vi "SyringePumpMain.vi"() -> ()   [LabVIEW 2016]
uses:
  <extravilib>/ChannelInstances/Tag-bool/Read With Abort.vi
  <extravilib>/ChannelInstances/Tag-bool/Write.vi
  <extravilib>/ChannelInstances/Tag-bool/Write With Abort.vi
  <extravilib>/ChannelInstances/Tag-bool/Instantiate.vi
  <extravilib>/ChannelInstances/Tag-bool/EndpointRead.vi
  <extravilib>/ChannelInstances/Tag-bool/Endpoint.vi
  <instrlib>/KD Scientific Legato 2XX Series/KD Scientific Legato 2XX Series.lvlib
  <extravilib>/ChannelInstances/Tag-bool.lvlib
panel:
  in  "Pause loop":bool
  in  "Infusion Rate \nUnits":u32(ring)=3 items=["ml/hr", "ml/min", "ul/hr", "ul/min", "ul/sec", "nl/sec"]
  out "Output infusion rate":string
  in  "Set infusion rate":bool
  in  "Infusion rate":dbl=2.0
  out "Output infusion volume":string
  in  "Set infusion volume":bool
  in  "Infusion \nVolume":i32=100
  in  "Infusion \nVolume unit":u16(ring) items=["µL", "nL", "mL"]
  out "Time remaining":dbl format="%<%H:%M:%S>t"
  out "Target reached?":bool
  out "Infusing?":bool
  out "Del. volume":string="0 nl"
  out "Path":path
  in  "Withdraw Rate \nUnits":u32(ring)=3 items=["ml/hr", "ml/min", "ul/hr", "ul/min", "ul/sec", "nl/sec"]
  out "Output withdraw rate":string
  in  "Set withdraw rate":bool
  in  "Withdraw rate":dbl=2.0
  out "Output withdraw volume":string
  in  "Set withdraw volume":bool
  in  "Withdraw \nVolume":i32=100
  in  "Withdraw \nVolume unit":u16(ring) items=["µL", "nL", "mL"]
  in  "Infuse":bool=TRUE
  in  "Withdraw":bool
  in  "Save Configuration":bool
  in  "Reset":bool
  in  "Start/Stop":bool
  in  "stop":bool
  in  "Syringe Volume Unit":u16(ring) items=["µL", "nL", "mL"]
  out "Output syringe volume":string
  in  "Set syringe volume":bool
  in  "Syringe Volume":i32=30 min=0 max=100 step=1
  out "Output force":string
  in  "Set force":bool
  in  "Current Force":i32=30 min=0 max=100 step=1
  out "Output syringe diameter":string
  in  "Set syringe diameter":bool
  in  "Syringe Diameter (mm)":dbl=4.86 min=0.01 max=49.99 step=0.01 format="%.2g"
  out "VISA resource":refnum<visa-resource-name>
  # "Syringe Volume"
  # "Force"
  # "Infusion rate"
  # "Infusion volume"
  # "Infusing:"
  # "Time remaining:"
  # "Volume delivered:"
  # "Target reached:"
  # "Withdraw rate"
  # "Withdraw volume"
  # "Syringe Diameter"
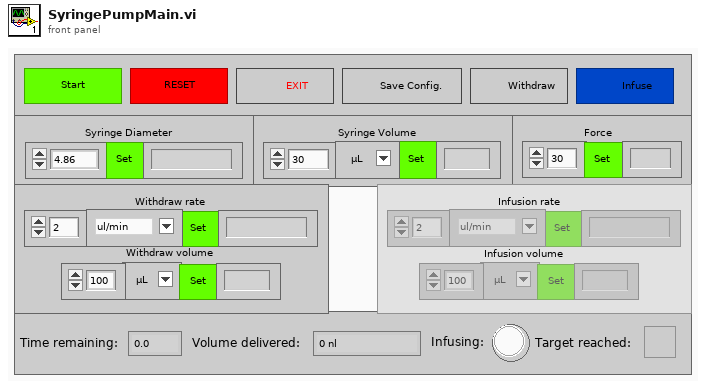
[diagram p1: front panel]
types:
  T1 = enum8{"Enabled", "Disabled", "Disabled and Grayed Out"}
  T2 = enum32{"invalid app kind", "Development System", "Run Time System", "Student Edition", "Embedded LabVIEW", "Evaluation", "Custom"}
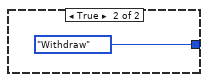
[diagram p4: hidden frame]
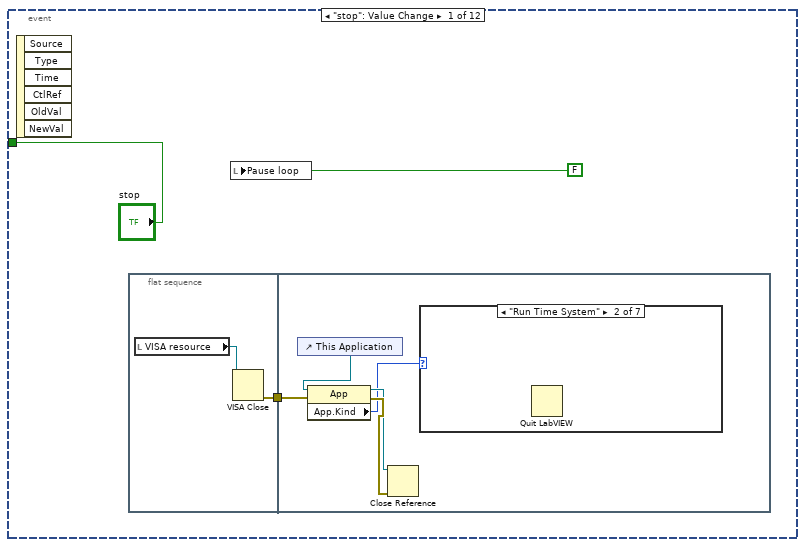
[diagram p6: hidden frame]
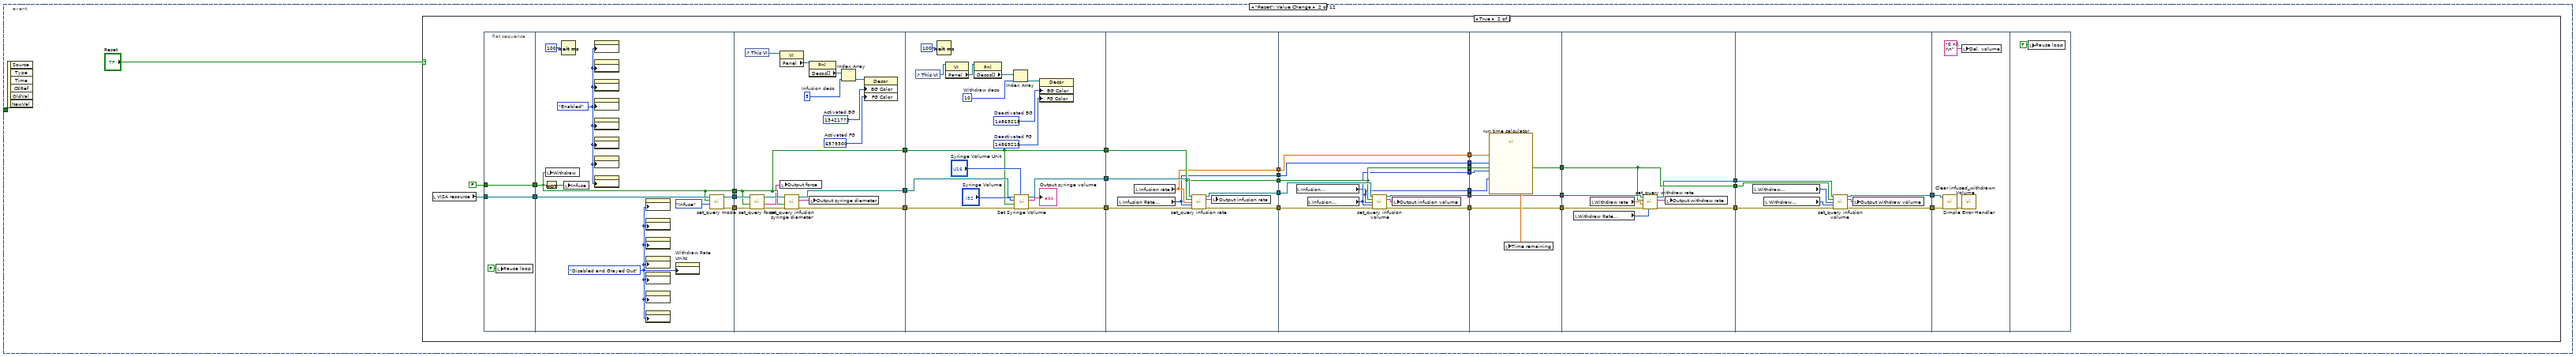
[diagram p13: hidden frame]
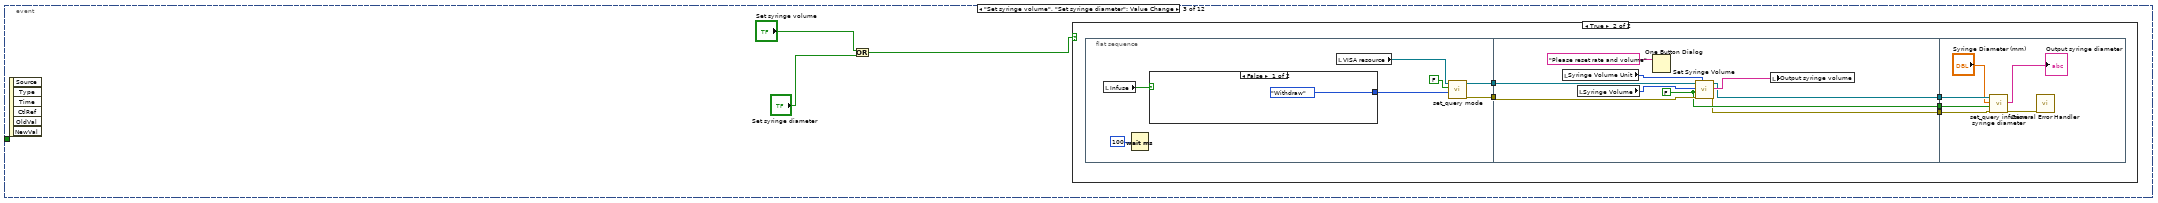
[diagram p15: hidden frame]
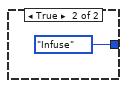
[diagram p17: hidden frame]
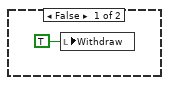
[diagram p18: hidden frame]
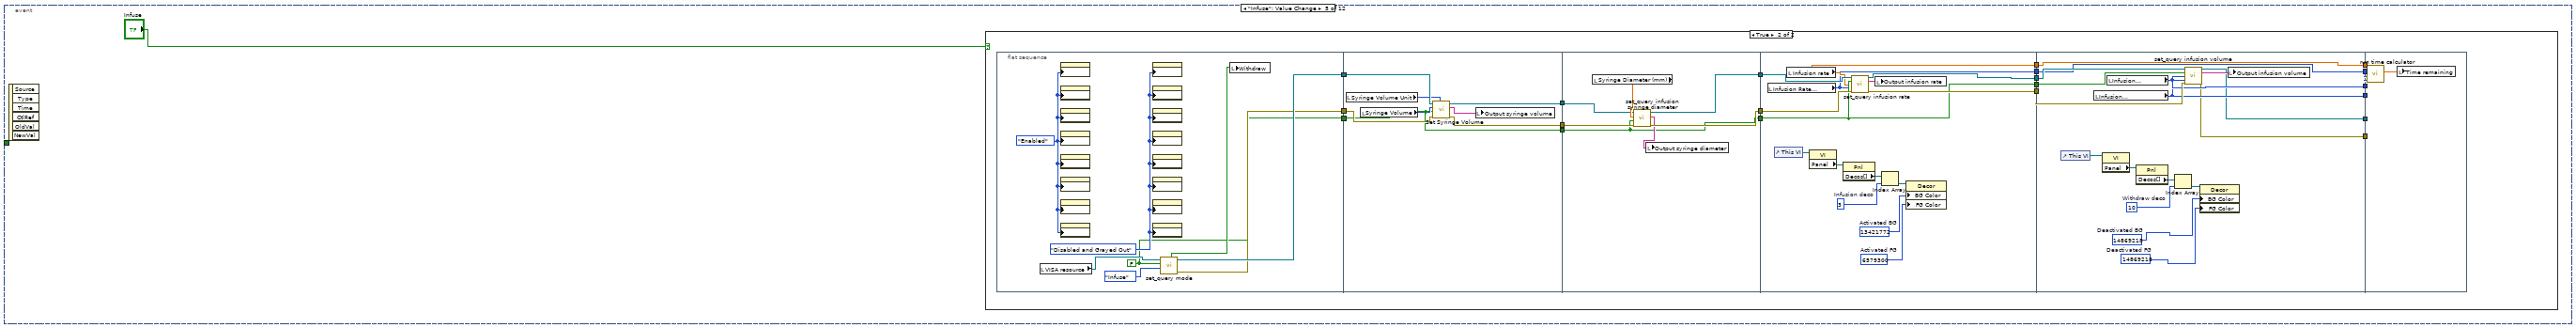
[diagram p19: hidden frame]
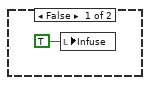
[diagram p20: hidden frame]
diagram:
  n1 = flat-sequence "Initialization sequence" {
    tunnel: [w39] -> w11
    tunnel: [w50] -> w32
    tunnel: [w73] -> w31
    tunnel: [w60] -> w30
    tunnel: [w72] -> w28
    tunnel: [w63] -> w26
    tunnel: [w55] -> w22
    tunnel: [w54] -> w14
    tunnel: [w53] -> w12
    tunnel: w11 -> [w51]
    tunnel: w32 -> [w99]
    tunnel: w31 -> [w96]
    tunnel: w30 -> [w103]
    tunnel: [w103] -> w29
    tunnel: w28 -> [w102]
    tunnel: [w102] -> w27
    tunnel: w26 -> [w101]
    tunnel: [w98] -> w25
    tunnel: [w97] -> w24
    tunnel: [w92] -> w23
    tunnel: w22 -> [w92]
    tunnel: w14 -> [w85]
    tunnel: [w84] -> w13
    tunnel: w12 -> [w84]
    tunnel: w29 -> [w118]
    tunnel: [w120] -> w38
    tunnel: w27 -> [w117]
    tunnel: [w116] -> w36
    tunnel: [w113] -> w35
    tunnel: w25 -> [w112]
    tunnel: w24 -> [w111]
    tunnel: w23 -> [w110]
    tunnel: [w110] -> w21
    tunnel: w13 -> [w104]
    tunnel: w38 -> [w129]
    tunnel: [w126] -> w37
    tunnel: w36 -> [w128]
    tunnel: w35 -> [w127]
    tunnel: [w127] -> w34
    tunnel: [w125] -> w33
    tunnel: w21 -> [w122]
    tunnel: [w122] -> w20
    tunnel: w37 -> [w138]
    tunnel: w34 -> [w135]
    tunnel: w33 -> [w139]
    tunnel: w20 -> [w141]
    tunnel: [w137] -> w19
    tunnel: [w140] -> w18
    tunnel: [w135] -> w17
    tunnel: [w141] -> w16
    tunnel: w19 -> [w146]
    tunnel: w18 -> [w147]
    tunnel: [w150] -> w10
    tunnel: w17 -> [w145]
    tunnel: w16 -> [w151]
    tunnel: [w145] -> w7
    tunnel: [w148] -> w4
    tunnel: [w151] -> w2
    tunnel: w10 -> [w158]
    tunnel: [w157] -> w8
    tunnel: w7 -> [w156]
    tunnel: [w156] -> w6
    tunnel: [w155] -> w5
    tunnel: w4 -> [w154]
    tunnel: [w153] -> w3
    tunnel: w2 -> [w153]
    tunnel: [w167] -> w9
    tunnel: w8 -> [w168]
    tunnel: w6 -> [w166]
    tunnel: w5 -> [w165]
    tunnel: w3 -> [w163]
    tunnel: [w163] -> w1
    tunnel: w9 -> [w177]
    tunnel: w1 -> [w176]
    frame #0 {
      n2 = control-ref of="This Application"() -> (w44:refnum<vi>)
      n3 = property class="App"(reference=w44) -> (reference out=w42:refnum<vi>, error out=w41:errorcluster, "App.Kind"=w43:T2)  [unwired: 1 in]
      n4 = control-ref of="This VI"() -> (w40:refnum<vi>)
      n5 = Close Reference(reference=w42, error in (no error)=w41) -> ()  [unwired: 1 out]
      n6 = invoke class="VI" method="Default Vals.Reinit All"(reference=w40) -> ()  [unwired: 2 in, 3 out]
      n7 = case shown="\"Run Time System\"" w43 {
        tunnel: [w45 w47 _ _ _ _ _] -> w39
        tunnel: w40 -> [w46 _ _ _ _ _ _]
        frame "Development System" {
          n8 = property class="VI"(reference=w46) -> ("Path"=w45:path)  [unwired: 1 in, 2 out]
        }
        frame "Run Time System" {
          n9 = call <userlib>:"Application Directory__ogtk.vi"() -> ("Application Directory (+ Relative)"=w49:path)  [unwired: 1 in]
          n10 = Build Path(base path=w49, name or relative path="Syringe Pump Controller\\") -> (appended path=w47:path)
        }
        frame "Student Edition" {
        }
        frame "Embedded LabVIEW" {
        }
        frame "Evaluation" {
        }
        frame "Custom" {
        }
        frame "invalid app kind" {
        }
      }
    }
    frame #1 {
      n11 = call "Config Reader.vi"("Path"=w51) -> ("Withdraw rate"=w56:dbl, "Withdraw \nVolume unit"=w58:u16, "Withdraw \nVolume"=w59:i32, "Default Current Force"=w72:i32, "Default Volume unit"=w69:u16, "Mode"=w65:string, "Withdraw Rate \nUnits"=w57:u32, "Default Syringe Volume Unit"=w66:u16, "Default Flow Rate Units (1:ml/min)"=w70:u32, "Default Volume"=w68:i32, "VISA Refnum out"=w50:refnum<visa-resource-name>, "Default Infusion rate"=w71:dbl, "Default Syringe Volume"=w67:i32, "Default Syringe Diameter (mm)"=w60:dbl, "error out"=w73:errorcluster)  [unwired: 4 in]
      n12 = local write "Current Force"(w72) -> ()
      n13 = local write "Infusion Rate \nUnits"(w70) -> ()
      n14 = local write "Infusion rate"(w71) -> ()
      n15 = local write "Syringe Diameter (mm)"(w60) -> ()
      n16 = local write "Syringe Volume"(w67) -> ()
      n17 = local write "Syringe Volume Unit"(w66) -> ()
      n18 = local write "Infusion \nVolume"(w68) -> ()
      n19 = local write "Infusion \nVolume unit"(w69) -> ()
      n20 = local write "Withdraw \nVolume"(w59) -> ()
      n21 = local write "Withdraw \nVolume unit"(w58) -> ()
      n22 = local write "Withdraw rate"(w56) -> ()
      n23 = local write "Withdraw Rate \nUnits"(w57) -> ()
      n24 = property class="Instr"(reference=w50, "General Settings:Timeout Value"=u32 10000) -> ()  [unwired: 1 in, 2 out]
      n25 = Equal?(x=w65, y="Infuse") -> (x = y?=w55:bool)
      n26 = case shown="True" w55 {
        tunnel: [enum16{"Withdraw", "Infuse"}."Withdraw" ("Mode Selector") enum16{"Withdraw", "Infuse"}."Infuse" ("Mode Selector")] -> w63
        tunnel: [T1."Disabled and Grayed Out" ("Disabled") T1."Enabled" ("Disabled")] -> w62
        tunnel: [T1."Enabled" ("Disabled") T1."Disabled and Grayed Out" ("Disabled")] -> w61
        tunnel: [w75 w79] -> w54
        tunnel: [w74 w80] -> w53
        frame False {
          w75 = 10  # Withdraw deco
          w74 = 3  # Infusion deco
        }
        frame True {
          w80 = 10  # Withdraw deco
          w79 = 3  # Infusion deco
        }
      }
      n27 = property on="Infusion \nVolume unit" class="Ring (strict)"("DisabledEnum"=w62) -> ()  [unwired: 2 in, 2 out]
      n28 = property on="Infusion \nVolume" class="DigNum (strict)"("DisabledEnum"=w62) -> ()  [unwired: 2 in, 2 out]
      n29 = property on="Infusion Rate \nUnits" class="Ring (strict)"("DisabledEnum"=w62) -> ()  [unwired: 2 in, 2 out]
      n30 = property on="Infusion rate" class="DigNum (strict)"("DisabledEnum"=w62) -> ()  [unwired: 2 in, 2 out]
      n31 = property on="Output infusion rate" class="Str"("DisabledEnum"=w62) -> ()  [unwired: 2 in, 2 out]
      n32 = property on="Output infusion volume" class="Str"("DisabledEnum"=w62) -> ()  [unwired: 2 in, 2 out]
      n33 = property on="Set infusion rate" class="Bool"("DisabledEnum"=w62) -> ()  [unwired: 2 in, 2 out]
      n34 = property on="Set infusion volume" class="Bool"("DisabledEnum"=w62) -> ()  [unwired: 2 in, 2 out]
      n35 = property on="Withdraw \nVolume unit" class="Ring (strict)"("DisabledEnum"=w61) -> ()  [unwired: 2 in, 2 out]
      n36 = property on="Withdraw \nVolume" class="DigNum (strict)"("DisabledEnum"=w61) -> ()  [unwired: 2 in, 2 out]
      n37 = property on="Withdraw Rate \nUnits" class="Ring (strict)"("DisabledEnum"=w61) -> ()  [unwired: 2 in, 2 out]
      n38 = property on="Withdraw rate" class="DigNum (strict)"("DisabledEnum"=w61) -> ()  [unwired: 2 in, 2 out]
      n39 = property on="Output withdraw rate" class="Str"("DisabledEnum"=w61) -> ()  [unwired: 2 in, 2 out]
      n40 = property on="Output withdraw volume" class="Str"("DisabledEnum"=w61) -> ()  [unwired: 2 in, 2 out]
      n41 = property on="Set withdraw volume" class="Bool"("DisabledEnum"=w61) -> ()  [unwired: 2 in, 2 out]
      n42 = property on="Set withdraw rate" class="Bool"("DisabledEnum"=w61) -> ()  [unwired: 2 in, 2 out]
      "Path" <- w51
    }
    frame #2 {
      w86 = u32 6579300  # Activated FG
      w87 = u32 13421772  # Activated BG
      n43 = control-ref of="This VI"() -> (w90:refnum<vi>)
      n44 = property class="VI"(reference=w90) -> ("Panel"=w91:refnum<vi>)  [unwired: 1 in, 2 out]
      n45 = call "set_query mode.vi"("error in (no error)"=w96, "Mode Selector"=w101, "Query?"=FALSE, "VISA resource name"=w99) -> ("error out"=w97:errorcluster, "Infuse?"=w94:bool, "VISA resource name out"=w98:refnum<visa-resource-name>, "Withdraw?"=w95:bool)  [unwired: 3 in, 1 out]
      n46 = local write "Withdraw"(w95) -> ()
      n47 = local write "Infuse"(w94) -> ()
      n48 = property class="Pnl"(reference=w91) -> ("Decos[]"=w89:refnum<vi>[])  [unwired: 1 in, 2 out]
      n49 = Index Array(array=w89, index=w85) -> (element=w88:refnum<vi>)
      n50 = Wait (ms)(milliseconds to wait=u32 100) -> ()  [unwired: 1 out]
      n51 = property class="Decor"(reference=w88, "BG Color"=w87, "FG Color"=w86) -> ()  [unwired: 1 in, 2 out]
    }
    frame #3 {
      w105 = u32 14869218  # Deactivated FG
      w106 = u32 14869218  # Deactivated BG
      w113 = FALSE ("Query?")
      n52 = property class="VI"() -> ("Panel"=w107:refnum<vi>)  [unwired: 2 in, 2 out]
      n53 = call "set_query force.vi"("error in (no error)"=w111, "Force Level (100 %)"=w117, "VISA resource name"=w112) -> ("error out"=w115:errorcluster, "Output force"=→"Output force":string, "VISA resource name out"=w114:refnum<visa-resource-name>)  [unwired: 6 in]
      n54 = property class="Pnl"(reference=w107) -> ("Decos[]"=w108:refnum<vi>[])  [unwired: 1 in, 2 out]
      n55 = Index Array(array=w108, index=w104) -> (element=w109:refnum<vi>)
      n56 = call "set_query infusion syringe diameter.vi"("error in (no error)"=w115, "Query?"=w113, "Syringe Diameter (20 mm)"=w118, "VISA resource name"=w114) -> ("error out"=w116:errorcluster, "Output syringe diameter"=w121:string, "VISA resource name out"=w120:refnum<visa-resource-name>)  [unwired: 5 in]
      n57 = local write "Output syringe diameter"(w121) -> ()
      n58 = property class="Decor"(reference=w109, "BG Color"=w106, "FG Color"=w105) -> ()  [unwired: 1 in, 2 out]
      n59 = control-ref of="This VI"() -> ()  [unwired: 1 out]
    }
    frame #4 {
      n60 = local read "Syringe Volume Unit"() -> (w130:u16)
      n61 = local read "Syringe Volume"() -> (w131:i32)
      n62 = call "Set Syringe Volume.vi"("Volume Units (0:ml)"=w130, "error in (no error)"=w128, "Query?"=w127, "Syringe volume"=w131, "VISA resource name"=w129) -> ("error out"=w125:errorcluster, "Output syringe volume"=w124:string, "VISA resource name out"=w126:refnum<visa-resource-name>)  [unwired: 4 in]
      n63 = local write "Output syringe volume"(w124) -> ()
      n64 = Wait (ms)(milliseconds to wait=u32 100) -> ()  [unwired: 1 out]
    }
    frame #5 {
      n65 = local read "Infusion Rate \nUnits"() -> (w133:u32)
      n66 = local read "Infusion rate"() -> (w134:dbl)
      n67 = call "set_query infusion rate.vi"("VISA resource name"=w138, "Query?"=w135, "Rate"=w134, "Flow Rate Units"=w133, "error in (no error)"=w139) -> ("VISA resource name out"=w137:refnum<visa-resource-name>, "Output infusion rate"=w136:string, "error out"=w140:errorcluster)  [unwired: 8 in]
      n68 = local write "Output infusion rate"(w136) -> ()
      n69 = Wait (ms)(milliseconds to wait=u32 100) -> ()  [unwired: 1 out]
    }
    frame #6 {
      n70 = local read "Infusion \nVolume unit"() -> (w143:u16)
      n71 = local read "Infusion \nVolume"() -> (w144:i32)
      n72 = call "set_query infusion volume.vi"("VISA resource name"=w146, "Query?"=w145, "Volume Units (0:ml)"=w143, "Volume"=w144, "error in (no error)"=w147) -> ("VISA resource name out"=w150:refnum<visa-resource-name>, "Output infusion volume"=w149:string, "error out"=w148:errorcluster)  [unwired: 8 in]
      n73 = local write "Output infusion volume"(w149) -> ()
      n74 = Wait (ms)(milliseconds to wait=u32 100) -> ()  [unwired: 1 out]
    }
    frame #7 {
      n75 = local read "Withdraw \nVolume unit"() -> (w160:u16)
      n76 = local read "Withdraw \nVolume"() -> (w161:i32)
      n77 = Wait (ms)(milliseconds to wait=u32 100) -> ()  [unwired: 1 out]
      n78 = call "set_query infusion volume.vi"("VISA resource name"=w158, "Query?"=w156, "Volume Units (0:ml)"=w160, "Volume"=w161, "error in (no error)"=w154) -> ("VISA resource name out"=w157:refnum<visa-resource-name>, "Output infusion volume"=w159:string, "error out"=w155:errorcluster)  [unwired: 8 in]
      n79 = local write "Output withdraw volume"(w159) -> ()
    }
    frame #8 {
      n80 = local read "Withdraw Rate \nUnits"() -> (w169:u32)
      n81 = local read "Withdraw rate"() -> (w170:dbl)
      n82 = call "set_query withdraw rate.vi"("Flow Rate Units"=w169, "error in (no error)"=w165, "Rate"=w170, "Query?"=w166, "VISA resource name"=w168) -> ("error out"=w164:errorcluster, "Output withdraw rate"=w171:string, "VISA resource name out"=w167:refnum<visa-resource-name>)  [unwired: 4 in]
      n83 = Wait (ms)(milliseconds to wait=u32 100) -> ()  [unwired: 1 out]
      n84 = local write "Output withdraw rate"(w171) -> ()
      n85 = call <vilib>:"Simple Error Handler.vi"("error in (no error)"=w164) -> ()  [unwired: 4 in, 5 out]
    }
    frame #9 {
      n86 = case shown="False" w176 {
        tunnel: [w181 w185] -> w175
        tunnel: [w180 w184] -> w174
        tunnel: [w179 w183] -> w173
        tunnel: [w182 w186] -> w172
        frame False {
          n87 = local read "Withdraw \nVolume unit"() -> (w179:u16)
          n88 = local read "Withdraw Rate \nUnits"() -> (w181:u32)
          n89 = local read "Withdraw \nVolume"() -> (w180:i32)
          n90 = local read "Withdraw rate"() -> (w182:dbl)
        }
        frame True {
          n91 = local read "Infusion \nVolume unit"() -> (w183:u16)
          n92 = local read "Infusion Rate \nUnits"() -> (w185:u32)
          n93 = local read "Infusion \nVolume"() -> (w184:i32)
          n94 = local read "Infusion rate"() -> (w186:dbl)
        }
      }
      n95 = call "run time calculator.vi"("Volume unit"=w173, "Volume"=w174, "Flow Rate Units (1:ml/min)"=w175, "Flow rate"=w172) -> ("time in seconds"=w178:dbl)  [unwired: 7 in]
      n96 = local write "Time remaining"(w178) -> ()
      "VISA resource" <- w177
    }
  }
  n97 = while {
    tunnel: [w187] -> w15
    stop <- w188 stop-if-true
    n98 = event shown="[3] \"Withdraw\": Value Change" {
      selector: _ -> [_ _ _ _ _ _ _ _ _ _ _ _]
      dyn-events: _ -> [_ _ _ _ _ _ _ _ _ _ _ _]
      timeout: _ -> [_ _ _ _ _ _ _ _ _ _ _ _]
      tunnel: ["stop" _ _ _ _ _ _ _ _ _ _ _] -> w189
      event "stop": Value Change {
        n99 = event-data() -> ()  [unwired: 1 in, 6 out]
        n100 = flat-sequence {
          tunnel: [w193] -> w190
          tunnel: w190 -> [w195]
          frame #0 {
            n101 = local read "VISA resource"() -> (w194:refnum<visa-resource-name>)
            n102 = VISA Close(VISA resource name=w194) -> (error out=w193:errorcluster)  [unwired: 1 in]
          }
          frame #1 {
            n103 = control-ref of="This Application"() -> (w196:refnum<vi>)
            n104 = property class="App"(reference=w196, error in=w195) -> (reference out=w198:refnum<vi>, error out=w199:errorcluster, "App.Kind"=w197:T2)
            n105 = Close Reference(reference=w198, error in (no error)=w199) -> ()  [unwired: 1 out]
            n106 = case shown="\"Run Time System\"" w197 {
              frame "Development System" {
              }
              frame "Run Time System" {
                n107 = Quit LabVIEW() -> ()  [unwired: 1 in]
              }
              frame "Student Edition" {
              }
              frame "Embedded LabVIEW" {
              }
              frame "Evaluation" {
              }
              frame "Custom" {
              }
              frame "invalid app kind" {
              }
            }
          }
        }
        n108 = local write "Pause loop"(FALSE ("Boolean")) -> ()
      }
      event "Reset": Value Change {
        n109 = event-data() -> ()  [unwired: 1 in, 6 out]
        n110 = case shown="True" "Reset" {
          frame False {
          }
          frame True {
            n111 = local read "VISA resource"() -> (w233:refnum<visa-resource-name>)
            n112 = flat-sequence {
              tunnel: FALSE ("Query?") -> [w235]
              tunnel: w233 -> [w236]
              tunnel: [w236] -> w206
              tunnel: [w235] -> w205
              tunnel: [w243] -> w222
              tunnel: [w237] -> w221
              tunnel: [w241] -> w220
              tunnel: w206 -> [w242]
              tunnel: w205 -> [w237]
              tunnel: [w258] -> w228
              tunnel: [w257] -> w226
              tunnel: [w256] -> w224
              tunnel: w222 -> [w259]
              tunnel: w221 -> [w257]
              tunnel: w220 -> [w253]
              tunnel: w228 -> [w273]
              tunnel: [w271] -> w227
              tunnel: w226 -> [w272]
              tunnel: [w272] -> w225
              tunnel: w224 -> [w274]
              tunnel: [w270] -> w223
              tunnel: w227 -> [w285]
              tunnel: [w284] -> w232
              tunnel: w225 -> [w283]
              tunnel: [w283] -> w230
              tunnel: [w281] -> w229
              tunnel: w223 -> [w282]
              tunnel: [w279] -> w217
              tunnel: [w278] -> w216
              tunnel: w232 -> [w295]
              tunnel: w230 -> [w292]
              tunnel: w229 -> [w294]
              tunnel: [w292] -> w219
              tunnel: w217 -> [w289]
              tunnel: w216 -> [w288]
              tunnel: [w291] -> w214
              tunnel: [w290] -> w210
              tunnel: [w289] -> w204
              tunnel: [w288] -> w203
              tunnel: [w287] -> w202
              tunnel: [w286] -> w201
              tunnel: w219 -> [w303]
              tunnel: [w303] -> w218
              tunnel: [w301] -> w215
              tunnel: w214 -> [w301]
              tunnel: w210 -> [w300]
              tunnel: [w300] -> w209
              tunnel: w204 -> [w299]
              tunnel: w203 -> [w298]
              tunnel: w202 -> [w297]
              tunnel: w201 -> [w296]
              tunnel: w218 -> [w307]
              tunnel: w215 -> [w308]
              tunnel: [w307] -> w213
              tunnel: [w306] -> w212
              tunnel: [w305] -> w211
              tunnel: w209 -> [w304]
              tunnel: w213 -> [w316]
              tunnel: w212 -> [w315]
              tunnel: w211 -> [w314]
              tunnel: [w313] -> w208
              tunnel: [w312] -> w207
              tunnel: w208 -> [w323]
              tunnel: w207 -> [w321]
              frame #0 {
                n113 = local write "Pause loop"(FALSE ("Boolean")) -> ()
              }
              frame #1 {
                w239 = T1."Disabled and Grayed Out" ("Disabled")
                w240 = T1."Enabled" ("Disabled")
                n114 = Not(x=w237) -> (.not. x?=w238:bool)
                n115 = local write "Withdraw"(w237) -> ()
                n116 = Wait (ms)(milliseconds to wait=u32 100) -> ()  [unwired: 1 out]
                n117 = local write "Infuse"(w238) -> ()
                n118 = property on="Set infusion rate" class="Bool"("DisabledEnum"=w240) -> ()  [unwired: 2 in, 2 out]
                n119 = property on="Output infusion volume" class="Str"("DisabledEnum"=w240) -> ()  [unwired: 2 in, 2 out]
                n120 = property on="Infusion \nVolume unit" class="Ring (strict)"("DisabledEnum"=w240) -> ()  [unwired: 2 in, 2 out]
                n121 = property on="Output infusion rate" class="Str"("DisabledEnum"=w240) -> ()  [unwired: 2 in, 2 out]
                n122 = property on="Infusion \nVolume" class="DigNum (strict)"("DisabledEnum"=w240) -> ()  [unwired: 2 in, 2 out]
                n123 = property on="Set infusion volume" class="Bool"("DisabledEnum"=w240) -> ()  [unwired: 2 in, 2 out]
                n124 = property on="Infusion rate" class="DigNum (strict)"("DisabledEnum"=w240) -> ()  [unwired: 2 in, 2 out]
                n125 = property on="Infusion Rate \nUnits" class="Ring (strict)"("DisabledEnum"=w240) -> ()  [unwired: 2 in, 2 out]
                n126 = property on="Output withdraw rate" class="Str"("DisabledEnum"=w239) -> ()  [unwired: 2 in, 2 out]
                n127 = property on="Withdraw \nVolume unit" class="Ring (strict)"("DisabledEnum"=w239) -> ()  [unwired: 2 in, 2 out]
                n128 = property on="Set withdraw rate" class="Bool"("DisabledEnum"=w239) -> ()  [unwired: 2 in, 2 out]
                n129 = property on="Withdraw \nVolume" class="DigNum (strict)"("DisabledEnum"=w239) -> ()  [unwired: 2 in, 2 out]
                n130 = property on="Withdraw rate" class="DigNum (strict)"("DisabledEnum"=w239) -> ()  [unwired: 2 in, 2 out]
                n131 = property on="Output withdraw volume" class="Str"("DisabledEnum"=w239) -> ()  [unwired: 2 in, 2 out]
                n132 = property on="Set withdraw volume" class="Bool"("DisabledEnum"=w239) -> ()  [unwired: 2 in, 2 out]
                n133 = property on="Withdraw Rate \nUnits" class="Ring (strict)"("DisabledEnum"=w239) -> ()  [unwired: 2 in, 2 out]
                n134 = call "set_query mode.vi"("Mode Selector"=enum16{"Withdraw", "Infuse"}."Infuse", "Query?"=w237, "VISA resource name"=w242) -> ("error out"=w241:errorcluster, "VISA resource name out"=w243:refnum<visa-resource-name>)  [unwired: 4 in, 3 out]
              }
              frame #2 {
                w252 = u32 6579300  # Activated FG
                w251 = u32 13421772  # Activated BG
                w246 = 3  # Infusion deco
                n135 = control-ref of="This VI"() -> (w248:refnum<vi>)
                n136 = call "set_query force.vi"("error in (no error)"=w253, "Query?"=w257, "VISA resource name"=w259) -> ("error out"=w260:errorcluster, "Output force"=w255:string, "VISA resource name out"=w261:refnum<visa-resource-name>)  [unwired: 6 in]
                n137 = property class="VI"(reference=w248) -> ("Panel"=w247:refnum<vi>)  [unwired: 1 in, 2 out]
                n138 = local write "Output force"(w255) -> ()
                n139 = call "set_query infusion syringe diameter.vi"("error in (no error)"=w260, "Query?"=w257, "VISA resource name"=w261) -> ("error out"=w256:errorcluster, "Output syringe diameter"=w254:string, "VISA resource name out"=w258:refnum<visa-resource-name>)  [unwired: 6 in]
                n140 = property class="Pnl"(reference=w247) -> ("Decos[]"=w249:refnum<vi>[])  [unwired: 1 in, 2 out]
                n141 = local write "Output syringe diameter"(w254) -> ()
                n142 = Index Array(array=w249, index=w246) -> (element=w250:refnum<vi>)
                n143 = property class="Decor"(reference=w250, "BG Color"=w251, "FG Color"=w252) -> ()  [unwired: 1 in, 2 out]
              }
              frame #3 {
                w268 = u32 14869218  # Deactivated FG
                w267 = u32 14869218  # Deactivated BG
                w266 = 10  # Withdraw deco
                n144 = control-ref of="This VI"() -> (w264:refnum<vi>)
                n145 = Wait (ms)(milliseconds to wait=u32 100) -> ()  [unwired: 1 out]
                n146 = property class="VI"(reference=w264) -> ("Panel"=w265:refnum<vi>)  [unwired: 1 in, 2 out]
                n147 = property class="Pnl"(reference=w265) -> ("Decos[]"=w263:refnum<vi>[])  [unwired: 1 in, 2 out]
                n148 = Index Array(array=w263, index=w266) -> (element=w262:refnum<vi>)
                n149 = call "Set Syringe Volume.vi"("Volume Units (0:ml)"="Syringe Volume Unit", "error in (no error)"=w274, "Query?"=w272, "Syringe volume"="Syringe Volume", "VISA resource name"=w273) -> ("error out"=w270:errorcluster, "Output syringe volume"=→"Output syringe volume":string, "VISA resource name out"=w271:refnum<visa-resource-name>)  [unwired: 4 in]
                n150 = property class="Decor"(reference=w262, "BG Color"=w267, "FG Color"=w268) -> ()  [unwired: 1 in, 2 out]
              }
              frame #4 {
                n151 = local read "Infusion Rate \nUnits"() -> (w278:u32)
                n152 = local read "Infusion rate"() -> (w279:dbl)
                n153 = call "set_query infusion rate.vi"("VISA resource name"=w285, "Query?"=w283, "Rate"=w279, "Flow Rate Units"=w278, "error in (no error)"=w282) -> ("VISA resource name out"=w284:refnum<visa-resource-name>, "Output infusion rate"=w280:string, "error out"=w281:errorcluster)  [unwired: 8 in]
                n154 = local write "Output infusion rate"(w280) -> ()
              }
              frame #5 {
                n155 = local read "Infusion \nVolume unit"() -> (w286:u16)
                n156 = local read "Infusion \nVolume"() -> (w287:i32)
                n157 = call "set_query infusion volume.vi"("VISA resource name"=w295, "Query?"=w292, "Volume Units (0:ml)"=w286, "Volume"=w287, "error in (no error)"=w294) -> ("VISA resource name out"=w291:refnum<visa-resource-name>, "Output infusion volume"=w293:string, "error out"=w290:errorcluster)  [unwired: 8 in]
                n158 = local write "Output infusion volume"(w293) -> ()
              }
              frame #6 {
                n159 = call "run time calculator.vi"("Volume unit"=w296, "Volume"=w297, "Flow Rate Units (1:ml/min)"=w298, "Flow rate"=w299) -> ("time in seconds"=w302:dbl)  [unwired: 7 in]
                n160 = local write "Time remaining"(w302) -> ()
              }
              frame #7 {
                n161 = local read "Withdraw Rate \nUnits"() -> (w309:u32)
                n162 = local read "Withdraw rate"() -> (w310:dbl)
                n163 = call "set_query withdraw rate.vi"("Flow Rate Units"=w309, "error in (no error)"=w304, "Rate"=w310, "Query?"=w307, "VISA resource name"=w308) -> ("error out"=w305:errorcluster, "Output withdraw rate"=w311:string, "VISA resource name out"=w306:refnum<visa-resource-name>)  [unwired: 4 in]
                n164 = local write "Output withdraw rate"(w311) -> ()
              }
              frame #8 {
                n165 = local read "Withdraw \nVolume unit"() -> (w317:u16)
                n166 = local read "Withdraw \nVolume"() -> (w318:i32)
                n167 = call "set_query infusion volume.vi"("VISA resource name"=w315, "Query?"=w316, "Volume Units (0:ml)"=w317, "Volume"=w318, "error in (no error)"=w314) -> ("VISA resource name out"=w313:refnum<visa-resource-name>, "Output infusion volume"=w319:string, "error out"=w312:errorcluster)  [unwired: 8 in]
                n168 = local write "Output withdraw volume"(w319) -> ()
              }
              frame #9 {
                n169 = call "Clear infused_withdrawn Volume.vi"("error in (no error)"=w321, "VISA resource name"=w323) -> ("error out"=w322:errorcluster)  [unwired: 8 in, 1 out]
                n170 = local write "Del. volume"("0 nl\r\n" ("Del. volume")) -> ()
                n171 = call <vilib>:"Simple Error Handler.vi"("error in (no error)"=w322) -> ()  [unwired: 4 in, 5 out]
              }
              frame #10 {
                n172 = local write "Pause loop"(TRUE ("Boolean")) -> ()
              }
            }
          }
        }
      }
      event "Set syringe volume", "Set syringe diameter": Value Change {
        n173 = event-data() -> ()  [unwired: 1 in, 6 out]
        n174 = Or(x="Set syringe volume", y="Set syringe diameter") -> (x .or. y?=w325:bool)
        n175 = case shown="True" w325 {
          frame False {
          }
          frame True {
            n176 = flat-sequence {
              tunnel: [w335] -> w332
              tunnel: [w334] -> w331
              tunnel: w332 -> [w346]
              tunnel: w331 -> [w345]
              tunnel: [w344] -> w330
              tunnel: [w343] -> w329
              tunnel: [w342] -> w328
              tunnel: w330 -> [w356]
              tunnel: w329 -> [w355]
              tunnel: w328 -> [w353]
              frame #0 {
                n177 = local read "Infuse"() -> (w337:bool)
                n178 = Wait (ms)(milliseconds to wait=u32 100) -> ()  [unwired: 1 out]
                n179 = case shown="False" w337 {
                  tunnel: [enum16{"Withdraw", "Infuse"}."Withdraw" ("Mode Selector") enum16{"Withdraw", "Infuse"}."Infuse" ("Mode Selector")] -> w339
                  frame False {
                  }
                  frame True {
                  }
                }
                n180 = local read "VISA resource"() -> (w338:refnum<visa-resource-name>)
                n181 = call "set_query mode.vi"("Mode Selector"=w339, "Query?"=FALSE, "VISA resource name"=w338) -> ("error out"=w335:errorcluster, "VISA resource name out"=w334:refnum<visa-resource-name>)  [unwired: 4 in, 3 out]
              }
              frame #1 {
                w343 = FALSE ("Query?")
                n182 = local read "Syringe Volume Unit"() -> (w349:u16)
                n183 = local read "Syringe Volume"() -> (w350:i32)
                n184 = One Button Dialog(message="Please reset rate and volume") -> ()  [unwired: 1 in, 1 out]
                n185 = call "Set Syringe Volume.vi"("Volume Units (0:ml)"=w349, "error in (no error)"=w346, "Query?"=w343, "Syringe volume"=w350, "VISA resource name"=w345) -> ("error out"=w342:errorcluster, "Output syringe volume"=w348:string, "VISA resource name out"=w344:refnum<visa-resource-name>)  [unwired: 4 in]
                n186 = local write "Output syringe volume"(w348) -> ()
              }
              frame #2 {
                n187 = call "set_query infusion syringe diameter.vi"("error in (no error)"=w353, "Query?"=w355, "Syringe Diameter (20 mm)"="Syringe Diameter (mm)", "VISA resource name"=w356) -> ("error out"=w354:errorcluster, "Output syringe diameter"=→"Output syringe diameter":string)  [unwired: 5 in, 1 out]
                n188 = call <vilib>:"General Error Handler.vi"("error in (no error)"=w354) -> ()  [unwired: 10 in, 5 out]
              }
            }
          }
        }
      }
      event "Withdraw": Value Change {
        n189 = event-data() -> ()  [unwired: 1 in, 6 out]
        n190 = case shown="True" "Withdraw" {
          frame False {
            n191 = local write "Withdraw"(TRUE ("Withdraw")) -> ()
          }
          frame True {
            n192 = flat-sequence {
              tunnel: [w381] -> w367
              tunnel: [w380] -> w366
              tunnel: [w379] -> w365
              tunnel: w367 -> [w387]
              tunnel: w366 -> [w385]
              tunnel: [w385] -> w363
              tunnel: w365 -> [w390]
              tunnel: [w389] -> w360
              tunnel: [w388] -> w359
              tunnel: [w397] -> w364
              tunnel: w363 -> [w393]
              tunnel: [w393] -> w362
              tunnel: [w398] -> w361
              tunnel: w360 -> [w399]
              tunnel: w359 -> [w396]
              tunnel: w364 -> [w414]
              tunnel: w362 -> [w409]
              tunnel: w361 -> [w413]
              tunnel: [w411] -> w376
              tunnel: [w410] -> w375
              tunnel: [w409] -> w374
              tunnel: [w408] -> w373
              tunnel: [w407] -> w372
              tunnel: w376 -> [w429]
              tunnel: w375 -> [w428]
              tunnel: w374 -> [w427]
              tunnel: w373 -> [w425]
              tunnel: [w425] -> w371
              tunnel: w372 -> [w424]
              tunnel: [w424] -> w370
              tunnel: [w423] -> w369
              tunnel: [w422] -> w368
              tunnel: w371 -> [w433]
              tunnel: w370 -> [w432]
              tunnel: w369 -> [w431]
              tunnel: w368 -> [w430]
              frame #0 {
                w377 = T1."Enabled" ("Disabled")
                w378 = T1."Disabled and Grayed Out" ("Disabled")
                w380 = FALSE ("Query?")
                n193 = local read "VISA resource"() -> (w383:refnum<visa-resource-name>)
                n194 = property on="Withdraw Rate \nUnits" class="Ring (strict)"("DisabledEnum"=w377) -> ()  [unwired: 2 in, 2 out]
                n195 = property on="Output withdraw rate" class="Str"("DisabledEnum"=w377) -> ()  [unwired: 2 in, 2 out]
                n196 = property on="Withdraw \nVolume unit" class="Ring (strict)"("DisabledEnum"=w377) -> ()  [unwired: 2 in, 2 out]
                n197 = property on="Set withdraw rate" class="Bool"("DisabledEnum"=w377) -> ()  [unwired: 2 in, 2 out]
                n198 = property on="Withdraw \nVolume" class="DigNum (strict)"("DisabledEnum"=w377) -> ()  [unwired: 2 in, 2 out]
                n199 = property on="Withdraw rate" class="DigNum (strict)"("DisabledEnum"=w377) -> ()  [unwired: 2 in, 2 out]
                n200 = property on="Output withdraw volume" class="Str"("DisabledEnum"=w377) -> ()  [unwired: 2 in, 2 out]
                n201 = property on="Set withdraw volume" class="Bool"("DisabledEnum"=w377) -> ()  [unwired: 2 in, 2 out]
                n202 = call "set_query mode.vi"("Mode Selector"=enum16{"Withdraw", "Infuse"}."Withdraw", "Query?"=w380, "VISA resource name"=w383) -> ("error out"=w379:errorcluster, "Infuse?"=w382:bool, "VISA resource name out"=w381:refnum<visa-resource-name>)  [unwired: 4 in, 2 out]
                n203 = property on="Set infusion rate" class="Bool"("DisabledEnum"=w378) -> ()  [unwired: 2 in, 2 out]
                n204 = property on="Output infusion volume" class="Str"("DisabledEnum"=w378) -> ()  [unwired: 2 in, 2 out]
                n205 = property on="Infusion \nVolume unit" class="Ring (strict)"("DisabledEnum"=w378) -> ()  [unwired: 2 in, 2 out]
                n206 = property on="Output infusion rate" class="Str"("DisabledEnum"=w378) -> ()  [unwired: 2 in, 2 out]
                n207 = property on="Infusion \nVolume" class="DigNum (strict)"("DisabledEnum"=w378) -> ()  [unwired: 2 in, 2 out]
                n208 = property on="Set infusion volume" class="Bool"("DisabledEnum"=w378) -> ()  [unwired: 2 in, 2 out]
                n209 = property on="Infusion rate" class="DigNum (strict)"("DisabledEnum"=w378) -> ()  [unwired: 2 in, 2 out]
                n210 = property on="Infusion Rate \nUnits" class="Ring (strict)"("DisabledEnum"=w378) -> ()  [unwired: 2 in, 2 out]
                n211 = local write "Infuse"(w382) -> ()
              }
              frame #1 {
                n212 = local read "Syringe Volume Unit"() -> (w392:u16)
                n213 = local read "Syringe Volume"() -> (w391:i32)
                n214 = call "Set Syringe Volume.vi"("Volume Units (0:ml)"=w392, "error in (no error)"=w390, "Query?"=w385, "Syringe volume"=w391, "VISA resource name"=w387) -> ("error out"=w389:errorcluster, "Output syringe volume"=w386:string, "VISA resource name out"=w388:refnum<visa-resource-name>)  [unwired: 4 in]
                n215 = local write "Output syringe volume"(w386) -> ()
              }
              frame #2 {
                n216 = local read "Syringe Diameter (mm)"() -> (w395:dbl)
                n217 = call "set_query infusion syringe diameter.vi"("error in (no error)"=w399, "Query?"=w393, "Syringe Diameter (20 mm)"=w395, "VISA resource name"=w396) -> ("error out"=w398:errorcluster, "Output syringe diameter"=w394:string, "VISA resource name out"=w397:refnum<visa-resource-name>)  [unwired: 5 in]
                n218 = local write "Output syringe diameter"(w394) -> ()
              }
              frame #3 {
                w406 = u32 14869218  # Deactivated FG
                w405 = u32 14869218  # Deactivated BG
                w404 = 3  # Infusion deco
                n219 = local read "Withdraw Rate \nUnits"() -> (w407:u32)
                n220 = control-ref of="This VI"() -> (w402:refnum<vi>)
                n221 = local read "Withdraw rate"() -> (w408:dbl)
                n222 = property class="VI"(reference=w402) -> ("Panel"=w403:refnum<vi>)  [unwired: 1 in, 2 out]
                n223 = property class="Pnl"(reference=w403) -> ("Decos[]"=w401:refnum<vi>[])  [unwired: 1 in, 2 out]
                n224 = call "set_query withdraw rate.vi"("Flow Rate Units"=w407, "error in (no error)"=w413, "Rate"=w408, "Query?"=w409, "VISA resource name"=w414) -> ("error out"=w410:errorcluster, "Output withdraw rate"=w412:string, "VISA resource name out"=w411:refnum<visa-resource-name>)  [unwired: 4 in]
                n225 = Index Array(array=w401, index=w404) -> (element=w400:refnum<vi>)
                n226 = local write "Output withdraw rate"(w412) -> ()
                n227 = property class="Decor"(reference=w400, "BG Color"=w405, "FG Color"=w406) -> ()  [unwired: 1 in, 2 out]
              }
              frame #4 {
                w415 = u32 6579300  # Activated FG
                w416 = u32 13421772  # Activated BG
                w421 = 10  # Withdraw deco
                n228 = local read "Withdraw \nVolume unit"() -> (w422:u16)
                n229 = local read "Withdraw \nVolume"() -> (w423:i32)
                n230 = control-ref of="This VI"() -> (w419:refnum<vi>)
                n231 = property class="VI"(reference=w419) -> ("Panel"=w420:refnum<vi>)  [unwired: 1 in, 2 out]
                n232 = property class="Pnl"(reference=w420) -> ("Decos[]"=w418:refnum<vi>[])  [unwired: 1 in, 2 out]
                n233 = call "set_query infusion volume.vi"("VISA resource name"=w429, "Query?"=w427, "Volume Units (0:ml)"=w422, "Volume"=w423, "error in (no error)"=w428) -> ("Output infusion volume"=w426:string)  [unwired: 8 in, 2 out]
                n234 = Index Array(array=w418, index=w421) -> (element=w417:refnum<vi>)
                n235 = local write "Output withdraw volume"(w426) -> ()
                n236 = property class="Decor"(reference=w417, "BG Color"=w416, "FG Color"=w415) -> ()  [unwired: 1 in, 2 out]
              }
              frame #5 {
                n237 = call "run time calculator.vi"("Volume unit"=w430, "Volume"=w431, "Flow Rate Units (1:ml/min)"=w432, "Flow rate"=w433) -> ("time in seconds"=w434:dbl)  [unwired: 7 in]
                n238 = local write "Time remaining"(w434) -> ()
              }
            }
          }
        }
      }
      event "Infuse": Value Change {
        n239 = event-data() -> ()  [unwired: 1 in, 6 out]
        n240 = case shown="True" "Infuse" {
          frame False {
            n241 = local write "Infuse"(TRUE ("Infuse")) -> ()
          }
          frame True {
            n242 = flat-sequence {
              tunnel: [w459] -> w445
              tunnel: [w458] -> w444
              tunnel: [w457] -> w443
              tunnel: w445 -> [w472]
              tunnel: w444 -> [w469]
              tunnel: w443 -> [w465]
              tunnel: [w467] -> w439
              tunnel: [w466] -> w438
              tunnel: [w465] -> w437
              tunnel: [w476] -> w442
              tunnel: [w475] -> w441
              tunnel: [w473] -> w440
              tunnel: w439 -> [w478]
              tunnel: w438 -> [w477]
              tunnel: w437 -> [w473]
              tunnel: w442 -> [w494]
              tunnel: [w493] -> w456
              tunnel: w441 -> [w492]
              tunnel: [w491] -> w455
              tunnel: w440 -> [w490]
              tunnel: [w490] -> w454
              tunnel: [w488] -> w453
              tunnel: [w487] -> w451
              tunnel: w456 -> [w511]
              tunnel: w455 -> [w510]
              tunnel: w454 -> [w509]
              tunnel: w453 -> [w507]
              tunnel: [w507] -> w452
              tunnel: w451 -> [w506]
              tunnel: [w506] -> w450
              tunnel: [w505] -> w449
              tunnel: [w504] -> w448
              tunnel: [w496] -> w447
              tunnel: [w495] -> w446
              tunnel: w452 -> [w516]
              tunnel: w450 -> [w515]
              tunnel: w449 -> [w514]
              tunnel: w448 -> [w513]
              tunnel: w447 -> [_]
              tunnel: w446 -> [_]
              frame #0 {
                w461 = T1."Enabled" ("Disabled")
                w462 = T1."Disabled and Grayed Out" ("Disabled")
                w457 = FALSE ("Query?")
                n243 = local read "VISA resource"() -> (w460:refnum<visa-resource-name>)
                n244 = property on="Set infusion volume" class="Bool"("DisabledEnum"=w461) -> ()  [unwired: 2 in, 2 out]
                n245 = property on="Infusion \nVolume unit" class="Ring (strict)"("DisabledEnum"=w461) -> ()  [unwired: 2 in, 2 out]
                n246 = property on="Output infusion rate" class="Str"("DisabledEnum"=w461) -> ()  [unwired: 2 in, 2 out]
                n247 = property on="Infusion Rate \nUnits" class="Ring (strict)"("DisabledEnum"=w461) -> ()  [unwired: 2 in, 2 out]
                n248 = property on="Infusion \nVolume" class="DigNum (strict)"("DisabledEnum"=w461) -> ()  [unwired: 2 in, 2 out]
                n249 = property on="Set infusion rate" class="Bool"("DisabledEnum"=w461) -> ()  [unwired: 2 in, 2 out]
                n250 = property on="Output infusion volume" class="Str"("DisabledEnum"=w461) -> ()  [unwired: 2 in, 2 out]
                n251 = property on="Infusion rate" class="DigNum (strict)"("DisabledEnum"=w461) -> ()  [unwired: 2 in, 2 out]
                n252 = property on="Set withdraw rate" class="Bool"("DisabledEnum"=w462) -> ()  [unwired: 2 in, 2 out]
                n253 = property on="Withdraw \nVolume unit" class="Ring (strict)"("DisabledEnum"=w462) -> ()  [unwired: 2 in, 2 out]
                n254 = property on="Output withdraw volume" class="Str"("DisabledEnum"=w462) -> ()  [unwired: 2 in, 2 out]
                n255 = property on="Withdraw \nVolume" class="DigNum (strict)"("DisabledEnum"=w462) -> ()  [unwired: 2 in, 2 out]
                n256 = property on="Set withdraw volume" class="Bool"("DisabledEnum"=w462) -> ()  [unwired: 2 in, 2 out]
                n257 = property on="Withdraw rate" class="DigNum (strict)"("DisabledEnum"=w462) -> ()  [unwired: 2 in, 2 out]
                n258 = property on="Output withdraw rate" class="Str"("DisabledEnum"=w462) -> ()  [unwired: 2 in, 2 out]
                n259 = property on="Withdraw Rate \nUnits" class="Ring (strict)"("DisabledEnum"=w462) -> ()  [unwired: 2 in, 2 out]
                n260 = call "set_query mode.vi"("Mode Selector"=enum16{"Withdraw", "Infuse"}."Infuse", "Query?"=w457, "VISA resource name"=w460) -> ("error out"=w458:errorcluster, "VISA resource name out"=w459:refnum<visa-resource-name>, "Withdraw?"=w463:bool)  [unwired: 4 in, 2 out]
                n261 = local write "Withdraw"(w463) -> ()
              }
              frame #1 {
                n262 = local read "Syringe Volume Unit"() -> (w471:u16)
                n263 = local read "Syringe Volume"() -> (w470:i32)
                n264 = call "Set Syringe Volume.vi"("Volume Units (0:ml)"=w471, "error in (no error)"=w469, "Query?"=w465, "Syringe volume"=w470, "VISA resource name"=w472) -> ("error out"=w466:errorcluster, "Output syringe volume"=w468:string, "VISA resource name out"=w467:refnum<visa-resource-name>)  [unwired: 4 in]
                n265 = local write "Output syringe volume"(w468) -> ()
              }
              frame #2 {
                n266 = local read "Syringe Diameter (mm)"() -> (w479:dbl)
                n267 = call "set_query infusion syringe diameter.vi"("error in (no error)"=w477, "Query?"=w473, "Syringe Diameter (20 mm)"=w479, "VISA resource name"=w478) -> ("error out"=w475:errorcluster, "Output syringe diameter"=w474:string, "VISA resource name out"=w476:refnum<visa-resource-name>)  [unwired: 5 in]
                n268 = local write "Output syringe diameter"(w474) -> ()
              }
              frame #3 {
                w486 = u32 6579300  # Activated FG
                w485 = u32 13421772  # Activated BG
                w480 = 3  # Infusion deco
                n269 = local read "Infusion Rate \nUnits"() -> (w487:u32)
                n270 = control-ref of="This VI"() -> (w482:refnum<vi>)
                n271 = local read "Infusion rate"() -> (w488:dbl)
                n272 = property class="VI"(reference=w482) -> ("Panel"=w481:refnum<vi>)  [unwired: 1 in, 2 out]
                n273 = property class="Pnl"(reference=w481) -> ("Decos[]"=w483:refnum<vi>[])  [unwired: 1 in, 2 out]
                n274 = call "set_query infusion rate.vi"("VISA resource name"=w494, "Query?"=w490, "Rate"=w488, "Flow Rate Units"=w487, "error in (no error)"=w492) -> ("VISA resource name out"=w493:refnum<visa-resource-name>, "Output infusion rate"=w489:string, "error out"=w491:errorcluster)  [unwired: 8 in]
                n275 = local write "Output infusion rate"(w489) -> ()
                n276 = Index Array(array=w483, index=w480) -> (element=w484:refnum<vi>)
                n277 = property class="Decor"(reference=w484, "BG Color"=w485, "FG Color"=w486) -> ()  [unwired: 1 in, 2 out]
              }
              frame #4 {
                w503 = u32 14869218  # Deactivated FG
                w502 = u32 14869218  # Deactivated BG
                w501 = 10  # Withdraw deco
                n278 = control-ref of="This VI"() -> (w499:refnum<vi>)
                n279 = local read "Infusion \nVolume unit"() -> (w504:u16)
                n280 = property class="VI"(reference=w499) -> ("Panel"=w500:refnum<vi>)  [unwired: 1 in, 2 out]
                n281 = local read "Infusion \nVolume"() -> (w505:i32)
                n282 = property class="Pnl"(reference=w500) -> ("Decos[]"=w498:refnum<vi>[])  [unwired: 1 in, 2 out]
                n283 = Index Array(array=w498, index=w501) -> (element=w497:refnum<vi>)
                n284 = call "set_query infusion volume.vi"("VISA resource name"=w511, "Query?"=w509, "Volume Units (0:ml)"=w504, "Volume"=w505, "error in (no error)"=w510) -> ("VISA resource name out"=w496:refnum<visa-resource-name>, "Output infusion volume"=w508:string, "error out"=w495:errorcluster)  [unwired: 8 in]
                n285 = property class="Decor"(reference=w497, "BG Color"=w502, "FG Color"=w503) -> ()  [unwired: 1 in, 2 out]
                n286 = local write "Output infusion volume"(w508) -> ()
              }
              frame #5 {
                n287 = call "run time calculator.vi"("Volume unit"=w513, "Volume"=w514, "Flow Rate Units (1:ml/min)"=w515, "Flow rate"=w516) -> ("time in seconds"=w512:dbl)  [unwired: 7 in]
                n288 = local write "Time remaining"(w512) -> ()
              }
            }
          }
        }
      }
      event "Set infusion rate": Value Change {
        n289 = event-data() -> ()  [unwired: 1 in, 6 out]
        n290 = case shown="True" "Set infusion rate" {
          frame False {
          }
          frame True {
            n291 = local read "VISA resource"() -> (w524:refnum<visa-resource-name>)
            n292 = local read "Infusion \nVolume unit"() -> (w518:u16)
            n293 = local read "Infusion \nVolume"() -> (w519:i32)
            n294 = call "run time calculator.vi"("Volume unit"=w518, "Volume"=w519, "Flow Rate Units (1:ml/min)"="Infusion Rate \nUnits", "Flow rate"="Infusion rate") -> ("time in seconds"=→"Time remaining":dbl)  [unwired: 7 in]
            n295 = call "set_query infusion rate.vi"("VISA resource name"=w524, "Query?"=FALSE, "Rate"="Infusion rate", "Flow Rate Units"="Infusion Rate \nUnits") -> ("Output infusion rate"=→"Output infusion rate":string, "error out"=w523:errorcluster)  [unwired: 9 in, 1 out]
            n296 = call <vilib>:"Simple Error Handler.vi"("error in (no error)"=w523) -> ()  [unwired: 4 in, 5 out]
          }
        }
      }
      event "Set infusion volume": Value Change {
        n297 = event-data() -> ()  [unwired: 1 in, 6 out]
        n298 = case shown="True" "Set infusion volume" {
          frame False {
          }
          frame True {
            n299 = local read "Infusion Rate \nUnits"() -> (w528:u32)
            n300 = local read "VISA resource"() -> (w535:refnum<visa-resource-name>)
            n301 = local read "Infusion rate"() -> (w529:dbl)
            n302 = call "run time calculator.vi"("Volume unit"="Infusion \nVolume unit", "Volume"="Infusion \nVolume", "Flow Rate Units (1:ml/min)"=w528, "Flow rate"=w529) -> ("time in seconds"=w532:dbl)  [unwired: 7 in]
            n303 = local write "Time remaining"(w532) -> ()
            n304 = call "set_query infusion volume.vi"("VISA resource name"=w535, "Query?"=FALSE, "Volume Units (0:ml)"="Infusion \nVolume unit", "Volume"="Infusion \nVolume") -> ("Output infusion volume"=→"Output infusion volume":string)  [unwired: 9 in, 2 out]
          }
        }
      }
      event "Set withdraw rate": Value Change {
        n305 = event-data() -> ()  [unwired: 1 in, 6 out]
        n306 = case shown="True" "Set withdraw rate" {
          frame False {
          }
          frame True {
            n307 = local read "VISA resource"() -> (w541:refnum<visa-resource-name>)
            n308 = local read "Withdraw \nVolume unit"() -> (w543:u16)
            n309 = local read "Withdraw \nVolume"() -> (w544:i32)
            n310 = call "set_query withdraw rate.vi"("Flow Rate Units"="Withdraw Rate \nUnits", "Rate"="Withdraw rate", "Query?"=FALSE, "VISA resource name"=w541) -> ("Output withdraw rate"=→"Output withdraw rate":string)  [unwired: 5 in, 2 out]
            n311 = call "run time calculator.vi"("Volume unit"=w543, "Volume"=w544, "Flow Rate Units (1:ml/min)"="Withdraw Rate \nUnits", "Flow rate"="Withdraw rate") -> ("time in seconds"=w542:dbl)  [unwired: 7 in]
            n312 = local write "Time remaining"(w542) -> ()
          }
        }
      }
      event "Set withdraw volume": Value Change {
        n313 = event-data() -> ()  [unwired: 1 in, 6 out]
        n314 = case shown="True" "Set withdraw volume" {
          frame False {
          }
          frame True {
            n315 = local read "VISA resource"() -> (w552:refnum<visa-resource-name>)
            n316 = local read "Withdraw Rate \nUnits"() -> (w548:u32)
            n317 = local read "Withdraw rate"() -> (w549:dbl)
            n318 = call "run time calculator.vi"("Volume unit"="Withdraw \nVolume unit", "Volume"="Withdraw \nVolume", "Flow Rate Units (1:ml/min)"=w548, "Flow rate"=w549) -> ("time in seconds"=w550:dbl)  [unwired: 7 in]
            n319 = call "set_query infusion volume.vi"("VISA resource name"=w552, "Query?"=FALSE, "Volume Units (0:ml)"="Withdraw \nVolume unit", "Volume"="Withdraw \nVolume") -> ("Output infusion volume"=→"Output withdraw volume":string)  [unwired: 9 in, 2 out]
            n320 = local write "Time remaining"(w550) -> ()
          }
        }
      }
      event "Save Configuration": Value Change {
        n321 = event-data() -> ()  [unwired: 1 in, 6 out]
        n322 = case shown="True" "Save Configuration" {
          frame False {
          }
          frame True {
            n323 = local read "Path"() -> (w555:path)
            n324 = local read "Syringe Diameter (mm)"() -> (w559:dbl)
            n325 = local read "Withdraw \nVolume unit"() -> (w564:u16)
            n326 = local read "Infusion \nVolume unit"() -> (w568:u16)
            n327 = local read "Withdraw Rate \nUnits"() -> (w563:u32)
            n328 = local read "Syringe Volume Unit"() -> (w556:u16)
            n329 = local read "Infusion Rate \nUnits"() -> (w558:u32)
            n330 = local read "Withdraw \nVolume"() -> (w562:i32)
            n331 = local read "Infusion \nVolume"() -> (w567:i32)
            n332 = local read "Syringe Volume"() -> (w557:i32)
            n333 = local read "Withdraw rate"() -> (w565:dbl)
            n334 = local read "Current Force"() -> (w561:i32)
            n335 = local read "Infusion rate"() -> (w560:dbl)
            n336 = local read "Withdraw"() -> (w566:bool)
            n337 = call "ConfigWriter.vi"("Path"=w555, "Mode"=w566, "Syringe Volume"=w557, "Withdraw \nVolume unit"=w564, "Withdraw rate"=w565, "Withdraw Rate \nUnits"=w563, "Withdraw \nVolume"=w562, "Syringe Diameter (mm)"=w559, "Infusion rate"=w560, "Infusion Rate Units"=w558, "Infusion volume"=w567, "Infusion volume unit"=w568, "Current Force"=w561, "Syringe Volume Unit"=w556) -> ()  [unwired: 5 in, 1 out]
          }
        }
      }
      event "Set force": Value Change {
        n338 = event-data() -> ()  [unwired: 1 in, 6 out]
        n339 = case shown="True" "Set force" {
          frame False {
          }
          frame True {
            n340 = local read "VISA resource"() -> (w573:refnum<visa-resource-name>)
            n341 = call "set_query force.vi"("Query?"=FALSE, "Force Level (100 %)"="Current Force", "VISA resource name"=w573) -> ("error out"=w570:errorcluster, "Output force"=w571:string)  [unwired: 6 in, 1 out]
            n342 = call <vilib>:"Simple Error Handler.vi"("error in (no error)"=w570) -> ()  [unwired: 4 in, 5 out]
            n343 = local write "Output force"(w571) -> ()
          }
        }
      }
      event "Start/Stop": Value Change {
        n344 = event-data() -> ()  [unwired: 1 in, 6 out]
        n345 = local read "VISA resource"() -> (w576:refnum<visa-resource-name>)
        n346 = case shown="True" "Start/Stop" {
          tunnel: w576 -> [w583 w586]
          tunnel: [w579 w589] -> w577
          frame False {
            w578 = FALSE ("Query?")
            n347 = call <instrlib>:"Stop Pump.vi"("VISA resource name"=w583) -> ("error out"=w581:errorcluster, "VISA resource name out"=w582:refnum<visa-resource-name>)  [unwired: 9 in]
            n348 = local write "Infusing?"(w578) -> ()
            n349 = call "set_query backlight.vi"("error in (no error)"=w581, "Query?"=w578, "Backlight (100 %)"=u32 100 ("Force Level (100 %)"), "VISA resource name"=w582) -> ("error out"=w579:errorcluster)  [unwired: 5 in, 2 out]
          }
          frame True {
            n350 = call "set_query backlight.vi"("Query?"=FALSE, "Backlight (100 %)"=u32 100 ("Force Level (100 %)"), "VISA resource name"=w586) -> ("error out"=w587:errorcluster, "VISA resource name out"=w588:refnum<visa-resource-name>)  [unwired: 6 in, 1 out]
            n351 = call <instrlib>:"Start Pump.vi"("error in (no error)"=w587, "VISA resource name"=w588) -> ("error out"=w589:errorcluster)  [unwired: 8 in, 1 out]
          }
        }
        n352 = call <vilib>:"Simple Error Handler.vi"("error in (no error)"=w577) -> ()  [unwired: 4 in, 5 out]
      }
    }
    n353 = call <vilib>:"Share Stop Signal.vi"("set stop (F)"=w189, "channel"=w187) -> ("stop"=w188:bool)
  }
  n354 = while "Measurable measurement loop" {
    shift-right: [w597] -> _
    shift-left: _ -> [w599]
    tunnel: w15 -> [w592]
    stop <- w590 stop-if-true
    w596 = 1 items=["no exception", "cancel error on match", "set error on match"] ("[exception action] (none:0)")
    n355 = local read "VISA resource"() -> (w594:refnum<visa-resource-name>)
    n356 = local read "Start/Stop"() -> (w600:bool)
    n357 = case shown="True" w600 {
      tunnel: w594 -> [_ w619]
      tunnel: [w603 w613] -> w598
      tunnel: w599 -> [w603 w618]
      frame False {
      }
      frame True {
        w609 = FALSE
        n358 = local read "Withdraw"() -> (w604:bool)
        n359 = local read "Time remaining"() -> (w612:dbl)
        n360 = case shown="False" w604 {
          tunnel: [enum16{"Withdraw", "Infuse"}."Infuse" ("Mode Selector") enum16{"Withdraw", "Infuse"}."Withdraw" ("Mode Selector")] -> w605
          frame False {
          }
          frame True {
          }
        }
        n361 = Decrement(x=w612) -> (x-1=w611:dbl)
        n362 = local write "Time remaining"(w611) -> ()
        n363 = call "infusion measurables.vi"("VISA resource name"=w619, "VISA wait (msec)"=u32 1, "Time"=w609, "Flow rate"=w609, "Volume"=TRUE, "error in (no error)"=w618, "Mode Selector"=w605) -> ("VISA resource name out"=w616:refnum<visa-resource-name>, "Delivered volume"=→"Del. volume":string, "error out"=w617:errorcluster)  [unwired: 8 in, 2 out]
        n364 = call "Status check.vi"("error in (no error)"=w617, "VISA resource name"=w616) -> ("error out"=w614:errorcluster, "Target reached?"=→"Target reached?":bool, "Infusing?"=w607:bool, "VISA resource name out"=w615:refnum<visa-resource-name>)  [unwired: 4 in, 2 out]
        "Infusing?" <- w607
        n365 = case shown="False" w607 {
          tunnel: w615 -> [w626 _]
          tunnel: w614 -> [w625 w631]
          tunnel: [w624 w631] -> w613
          tunnel: w607 -> [w623 _]
          frame False {
            n366 = local write "Start/Stop"(w623) -> ()
            n367 = call <instrlib>:"Stop Pump.vi"("error in (no error)"=w625, "VISA resource name"=w626) -> ("error out"=w629:errorcluster, "VISA resource name out"=w630:refnum<visa-resource-name>)  [unwired: 8 in]
            n368 = call "set_query backlight.vi"("error in (no error)"=w629, "Query?"=FALSE, "Backlight (100 %)"=u32 100 ("Force Level (100 %)"), "VISA resource name"=w630) -> ("error out"=w624:errorcluster)  [unwired: 5 in, 2 out]
          }
          frame True {
          }
        }
      }
    }
    n369 = call <vilib>:"General Error Handler.vi"("error in (no error)"=w598, "[exception action] (none:0)"=w596, "[exception code]"=1073807339) -> ("error out"=w597:errorcluster)  [unwired: 8 in, 4 out]
    n370 = case shown="True" "Pause loop" {
      frame False {
      }
      frame True {
        n371 = while {
          stop <- w601 continue-if-true
          n372 = local read "Pause loop"() -> (w601:bool)
          n373 = Wait (ms)(milliseconds to wait=u32 10) -> ()  [unwired: 1 out]
        }
      }
    }
    n374 = call <extravilib>:"Read.vi"("channel"=w592) -> ("element"=w590:bool)  [unwired: 1 in, 1 out]
    n375 = Wait (ms)(milliseconds to wait=u32 1000) -> ()  [unwired: 1 out]
  }
